vi "trackBlobs.vi"(4 "WiFi Info":T3={"WiFi"={"SSID"="", "Key"=""}, "SystemLink"={"APIKey"="", "Tag"="", "Type"="STRING"}}, 6 "Output":enum16{"None", "UART", "SPI", "I2C", "WiFi"}(ring), 7 "ROI":T1, 8 "error in (no error)":errorcluster, 10 "Blob Params":T2={"Feature"=enum."cx", "Lab thresholds"="[10,90,-20,20,-20,20]", "Minimum Pixels"=100, "Minimum Area (box)"=100, "Merge"=TRUE, "Margin for merge"=10}, 11 "VISA Refnum in":refnum<visa-resource-name>) -> (0 "error out":errorcluster, 2 "Python Code":string, 3 "VISA Refnum out":refnum<visa-resource-name>)   [LabVIEW 2017]
uses:
  <userlib>/LabVIEWOpenMV/_subs/CameraSetup.ctl
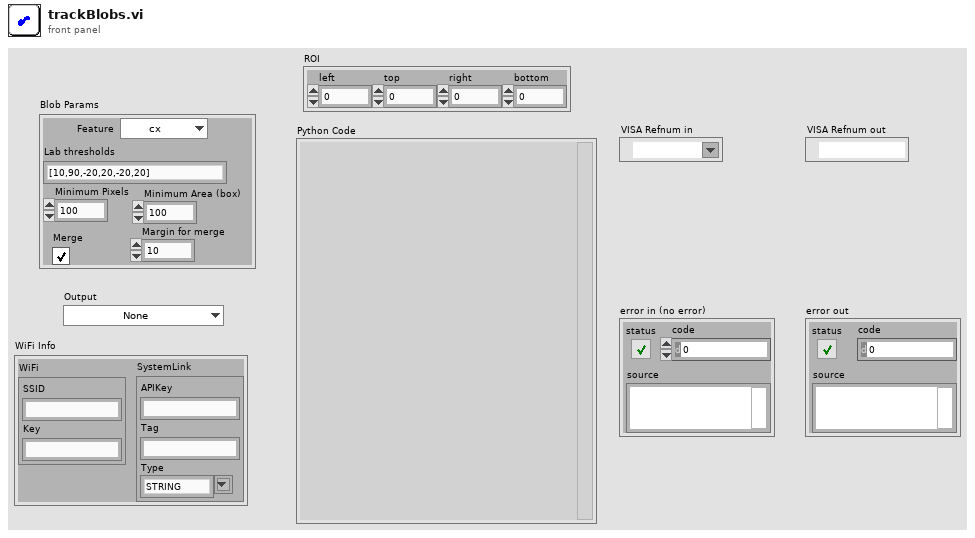
[diagram p1: front panel]
types:
  T1 = cluster{"left":i32, "top":i32, "right":i32, "bottom":i32}
  T2 = cluster{"Feature":enum16{"x", "y", "width", "height", "pixels", "cx", "cy", "rotation", "code", "count", "# blobs", "All parameters"}, "Lab thresholds":string, "Minimum Pixels":i16, "Minimum Area (box)":i16, "Merge":bool, "Margin for merge":i16}
  T3 = cluster{"WiFi":cluster{"SSID":string, "Key":string}, "SystemLink":cluster{"APIKey":string, "Tag":string, "Type":string}}
  T4 = typedef "CameraSetup.ctl" = cluster{"Format":enum16{"GRAYSCALE", "RGB565", "BAYER"}, "size":enum16{"QQQQVGA (40x30)", "QQQVGA (80x60)", "QQVGA (160x120)", "QVGA (320x240)", "VGA (640x480)", "LCD (128x160)", "B64x32 (64x32)", "B64x64", "B128x64", "B128x128"}, "Skip frames (ms)":u16, "autoGain":bool, "autoWhitebal":bool}
  T5 = enum16{"x", "y", "width", "height", "pixels", "cx", "cy", "rotation", "code", "count", "# blobs", "All parameters"}
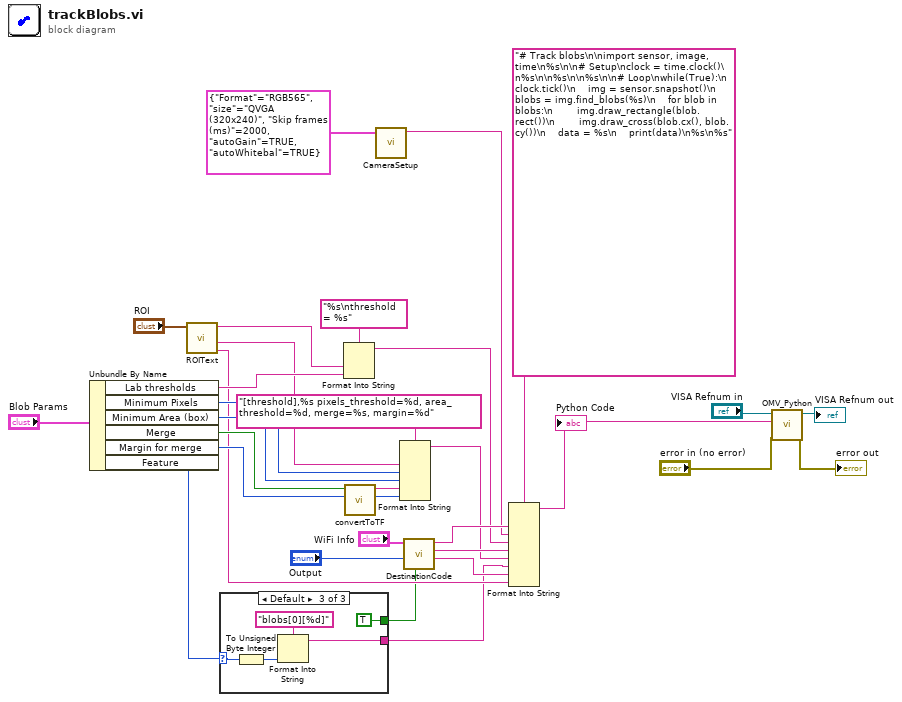
[diagram p0: block diagram]
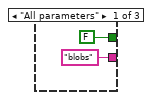
[diagram p2: hidden frame]
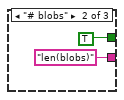
[diagram p3: hidden frame]
diagram:
  n1 = Unbundle By Name("Blob Params") -> ("Lab thresholds"=w15:string, "Minimum Pixels"=w13:i16, "Minimum Area (box)"=w12:i16, "Merge"=w10:bool, "Margin for merge"=w11:i16, "Feature"=w3:T5)
  n2 = call <userlib>:"ROIText.vi"("ROI"="ROI") -> ("draw"=w5:string, "with comma"=w4:string, "r"=w6:string)  [unwired: 7 in, 1 out]
  n3 = case shown="Default" w3 {
    selector: w3 -> [_ _ w40]
    tunnel: ["blobs" "len(blobs)" w38] -> w2
    tunnel: [FALSE TRUE TRUE] -> w1
    frame "All parameters" {
    }
    frame "# blobs" {
    }
    frame Default {
      n4 = To Unsigned Byte Integer(number=w40) -> (unsigned 8bit integer=w39:u8)
      n5 = Format Into String(format string="blobs[0][%d]", w39) -> (resulting string=w38:string)  [unwired: 2 in, 1 out]
    }
  }
  n6 = Format Into String(format string="%s\nthreshold = %s", w6, w15) -> (resulting string=w17:string)  [unwired: 2 in, 1 out]
  n7 = call <userlib>:"convertToTF.vi"("Boolean"=w10) -> ("Text"=w9:string)  [unwired: 10 in]
  n8 = call <userlib>:"CameraSetup.vi"("Camera Setup"=T4 {"Format"=enum."RGB565", "size"=enum."QVGA (320x240)", "Skip frames (ms)"=2000, "autoGain"=TRUE, "autoWhitebal"=TRUE}) -> ("String"=w25:string)  [unwired: 10 in]
  n9 = Format Into String(format string="[threshold],%s pixels_threshold=%d, area_threshold=%d, merge=%s, margin=%d", w4, w13, w12, w9, w11) -> (resulting string=w8:string)  [unwired: 2 in, 1 out]
  n10 = call <userlib>:"DestinationCode.vi"("Single number?"=w1, "Destination"="Output", "WiFi Info"="WiFi Info") -> ("Repeated call"=w28:string, "Setup"=w29:string, "Headers"=w26:string)  [unwired: 6 in]
  n11 = Format Into String(format string="# Track blobs\n\nimport sensor, image, time\n%s\n\n# Setup\nclock = time.clock()\n%s\n\n%s\n\n%s\n\n# Loop\nwhile(True):\n    clock.tick()\n    img = sensor.snapshot()\n    blobs = img.find_blobs(%s)\n    for blob in blobs:\n        img.draw_rectangle(blob.rect())\n        img.draw_cross(blob.cx(), blob.cy())\n    data = %s\n    print(data)\n%s\n%s" ("startCode"), w26, w25, w17, w29, w8, w2, w28, w5) -> (resulting string=w19:string)  [unwired: 2 in, 1 out]
  "Python Code" <- w19
  n12 = call <userlib>:"OMV_Python.vi"("error in (no error)"="error in (no error)", "Script"=w19, "VISA Refnum in"="VISA Refnum in") -> ("error out"=→"error out":errorcluster, "VISA Refnum out"=→"VISA Refnum out":refnum<visa-resource-name>)  [unwired: 7 in]
